vi "generate symbols.vi"(11 "M-ary":i32) -> (3 "Array":cdb[](array[numeric]))   [LabVIEW 2013]
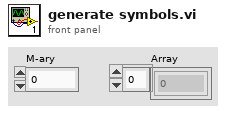
[diagram p1: front panel]
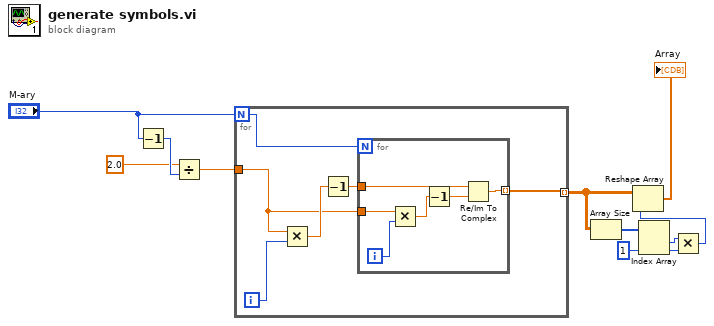
[diagram p0: block diagram]
diagram:
  n1 = Decrement(x="M-ary") -> (x-1=w3:i32)
  n2 = Divide(x=2.0, y=w3) -> (x/y=w4:dbl)
  n3 = for {
    N: "M-ary" -> [w12]
    tunnel: w4 -> [w15]
    tunnel: [w13] -> w6 mode=indexing
    i -> [w17]
    n4 = Multiply(x=w15, y=w17) -> (x*y=w16:dbl)
    n5 = Decrement(x=w16) -> (x-1=w14:dbl)
    n6 = for {
      N: w12 -> [_]
      tunnel: w14 -> [w19]
      tunnel: w15 -> [w22]
      tunnel: [w18] -> w13 mode=indexing
      i -> [w21]
      n7 = Multiply(x=w22, y=w21) -> (x*y=w23:dbl)
      n8 = Decrement(x=w23) -> (x-1=w20:dbl)
      n9 = Re/Im To Complex(1:w20, 2:w19) -> (0:w18:cdb)
    }
  }
  n10 = Array Size(array=w6) -> (size(s)=w7:i32[])
  n11 = Index Array(array=w7, index #2=1 ("index")) -> (element #1=w9:i32, element #2=w10:i32)  [unwired: 1 in]
  n12 = Multiply(x=w9, y=w10) -> (x*y=w11:i32)
  n13 = Reshape Array(w6, w11) -> (→"Array":cdb[])
